vi "Write Common Parameters to string.vi"(1 "Parameters - String":T1[](array[typedef]), 2 "Parameters - Numeric":T2[](array[typedef]), 3 "Script Parameters":map{string, string}(c390)) -> (0 "String":string)   [LabVIEW 2020, in "CIRCUS_uServices.lvlib" / "Run Utilities.lvlib" / "Optimiser Cell.lvclass"]
uses:
  Optimiser Cell.lvclass
  Optimise parameter - numeric.ctl
  Optimise parameter - string.ctl
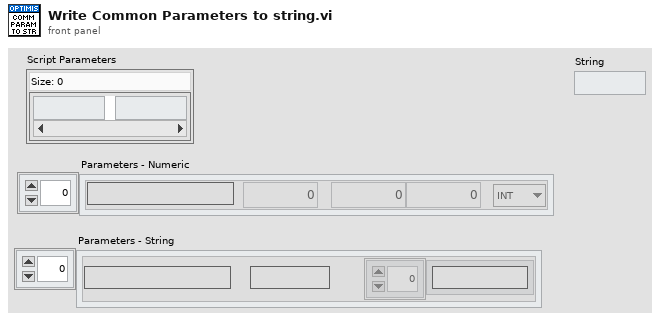
[diagram p1: front panel]
types:
  T1 = typedef "CIRCUS_uServices.lvlib/Run Utilities.lvlib/Optimiser Cell.lvclass/Optimise parameter - string.ctl" = cluster{"Name":string, "Start value":string, "Options":string[]}
  T2 = typedef "CIRCUS_uServices.lvlib/Run Utilities.lvlib/Optimiser Cell.lvclass/Optimise parameter - numeric.ctl" = cluster{"Name":string, "Start value":dbl, "From":dbl, "To":dbl, "dtype":enum16{"INT", "DBL"}}
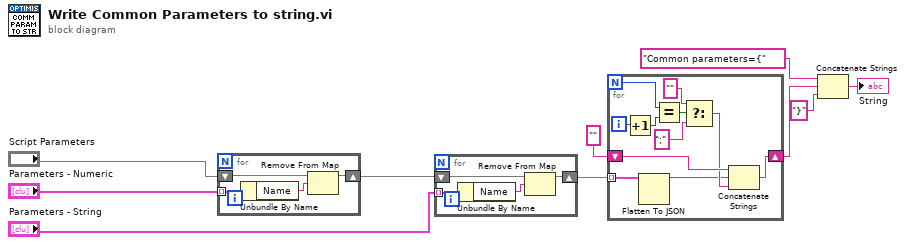
[diagram p0: block diagram]
diagram:
  n1 = for {
    shift-right: [w13] -> w10
    shift-left: "Script Parameters" -> [w14]
    tunnel: "Parameters - Numeric" -> [w12] mode=indexing
    n2 = Unbundle By Name(w12) -> ("Name"=w11:string)
    n3 = Remove From Map(10:w11, 11:w14) -> (3:w13:map{string, string})  [unwired: 2 out]
  }
  n4 = for {
    shift-right: [w17] -> w5
    shift-left: w10 -> [w18]
    tunnel: "Parameters - String" -> [w16] mode=indexing
    n5 = Unbundle By Name(w16) -> ("Name"=w15:string)
    n6 = Remove From Map(10:w15, 11:w18) -> (3:w17:map{string, string})  [unwired: 2 out]
  }
  n7 = for {
    N -> [w25]
    tunnel: w5 -> [w20] mode=indexing
    shift-right: [w28] -> w7
    shift-left: "" ("string") -> [w29]
    i -> [w27]
    n8 = Increment(x=w27) -> (x+1=w26:i32)
    n9 = Flatten To JSON(anything=w20) -> (JSON string=w19:string)  [unwired: 2 in, 1 out]
    n10 = Equal?(x=w25, y=w26) -> (x = y?=w24:bool)
    n11 = Select(t="" ("string"), s=w24, f=";") -> (s? t:f=w21:string)
    n12 = Concatenate Strings(w29, w19, w21) -> (w28:string)
  }
  n13 = Concatenate Strings("Common parameters={" ("string"), w7, "}" ("string")) -> (→"String":string)
